vi "Clear_Return List.vi"(8 "error in (no error)":errorcluster, 11 "InconsistentList in":refnum<class "NI_Robotics_InconsistentList.lvclass">) -> (0 "error out":errorcluster, 2 "nodes":refnum<data-value>[](array[refnum]), 3 "InconsistentList out":refnum<class "NI_Robotics_InconsistentList.lvclass">)   [LabVIEW 2017, in "NI_Robotics_InconsistentList.lvclass"]
uses:
  <vilib>/robotics/Navigation/shared/InconsistentList/NI_Robotics_InconsistentList.lvclass
  <vilib>/robotics/Navigation/shared/MapNode/AbstractDstarNode/NI_Robotics_AbstractDstarNode.lvclass
  <vilib>/robotics/Navigation/shared/InconsistentList/NI_Robotics_InconsistentList.lvclass/NI_Robotics_InconsistentList.ctl
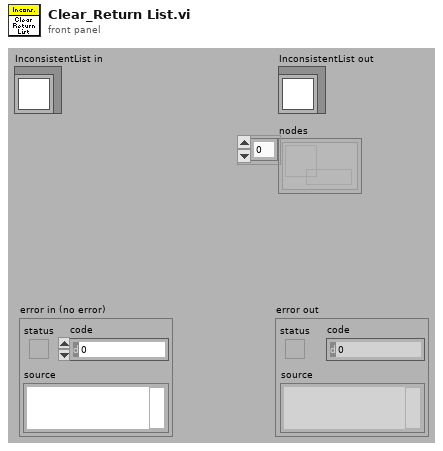
[diagram p1: front panel]
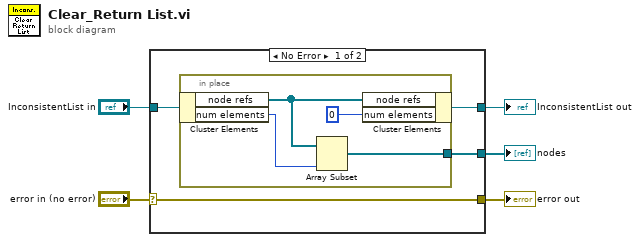
[diagram p0: block diagram]
diagram:
  n1 = case shown="No Error" "error in (no error)" {
    selector: "error in (no error)" -> [w8 w14]
    tunnel: "InconsistentList in" -> [w6 w15]
    tunnel: [w9 _] -> w1
    tunnel: [w7 w15] -> w4
    tunnel: [w8 w14] -> w2
    frame No Error {
      n2 = in-place {
        in-place-border: [w13] -> w9
        n3 = in-place-cluster #1(w6) -> ("node refs"=w12:refnum<data-value>[], "num elements"=w11:i32)
        n4 = Array Subset(array=w12, length=w11) -> (w13:refnum<data-value>[])  [unwired: 1 in]
        n5 = in-place-cluster #1("node refs"=w12, "num elements"=0) -> (w7:refnum<class "NI_Robotics_InconsistentList.lvclass">)
      }
    }
    frame Error {
    }
  }
  "InconsistentList out" <- w4
  "nodes" <- w1
  "error out" <- w2
